vi "BRig_dataCurrent_nReward_total_L.vi"() -> (2 "output_nReward_total_L":i32)   [LabVIEW 2014]
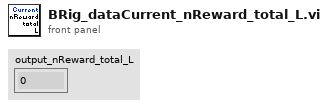
[diagram p1: front panel]
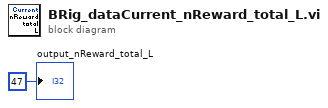
[diagram p0: block diagram]
diagram:
  "output_nReward_total_L" <- 47 ("output_iBlock")
